vi "ROI for multifit.vi"(9 "Cursor En Max":dbl, 10 "Cursor En Min":dbl, 11 "Spectrum In":cluster{"Locations":dbl[], "Amplitudes":dbl[]}={"Locations"=array[8192 elements], "Amplitudes"=array[8192 elements]}) -> (3 "Spectrum Reuced":cluster{"Array":dbl[], "Array":dbl[]})   [LabVIEW 2023]
panel:
  out "Spectrum":cluster{"Locations":dbl[], "Amplitudes":dbl[]}[](graph)
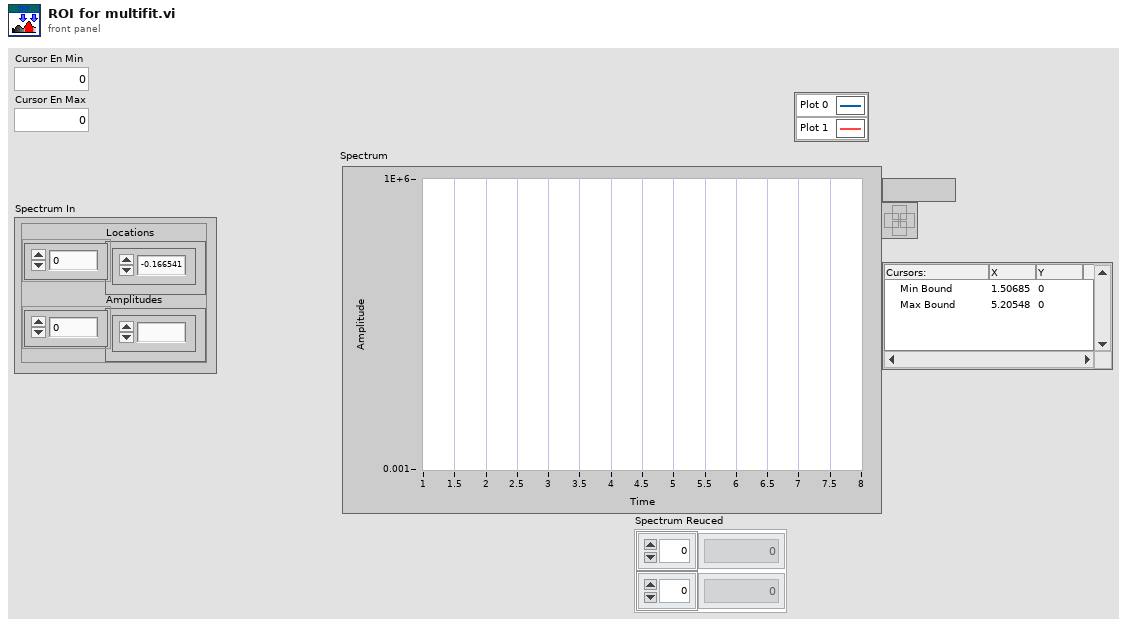
[diagram p1: front panel]
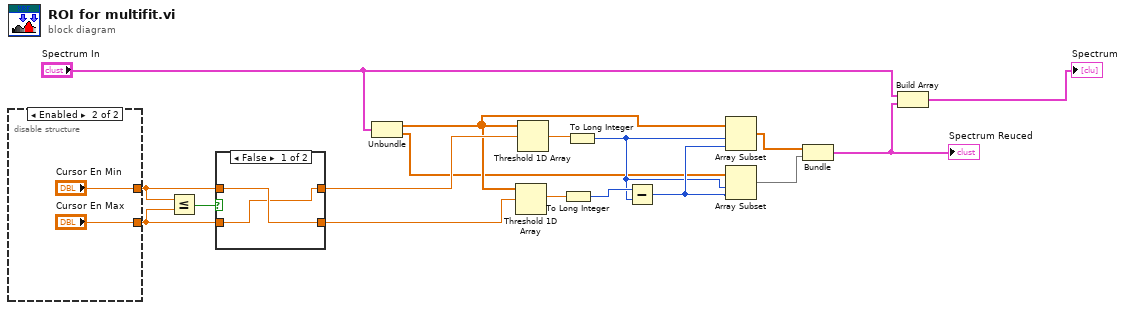
[diagram p0: block diagram]
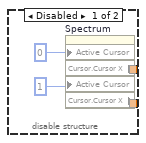
[diagram p2: hidden frame]
diagram:
  n1 = disable-structure shown="Enabled" {
    disable-tunnel: [w19 "Cursor En Min"] -> w16
    disable-tunnel: [w18 "Cursor En Max"] -> w15
    frame Disabled {
      n2 = property on="Spectrum" class="XYGraph (strict)"("Active Cursor"=u32 0, "Active Cursor"=u32 1) -> ("Cursor.Cursor X"=w19:dbl, "Cursor.Cursor X"=w18:dbl)  [unwired: 2 in, 2 out]
    }
    frame Enabled {
    }
  }
  n3 = Less Or Equal?(x=w16, y=w15) -> (x <= y?=w17:bool)
  n4 = case shown="False" w17 {
    tunnel: [w24 w27] -> w14
    tunnel: w16 -> [w25 w27]
    tunnel: [w25 w26] -> w13
    tunnel: w15 -> [w24 w26]
    frame False {
    }
    frame True {
    }
  }
  n5 = Unbundle("Spectrum In") -> ("Locations"=w7:dbl[], "Amplitudes"=w6:dbl[])
  n6 = Threshold 1D Array(2:w13, 3:w7) -> (0:w11:dbl)  [unwired: 1 in]
  n7 = Threshold 1D Array(2:w14, 3:w7) -> (0:w12:dbl)  [unwired: 1 in]
  n8 = To Long Integer(number=w11) -> (32bit integer=w10:i32)
  n9 = To Long Integer(number=w12) -> (32bit integer=w8:i32)
  n10 = Subtract(x=w10, y=w8) -> (x-y=w9:i32)
  n11 = Array Subset(array=w7, index=w8, length=w9) -> (w5:dbl[])
  n12 = Array Subset(array=w6, index=w8, length=w9) -> (w4:dbl[])
  n13 = Bundle(w5, w4) -> (w2:cluster{dbl[], dbl[]})  [unwired: 1 in]
  "Spectrum Reuced" <- w2
  n14 = Build Array("Spectrum In", w2) -> (→"Spectrum":cluster{"Locations":dbl[], "Amplitudes":dbl[]}[])
